vi "#0_MAV_MSG_HEARTBEAT.vi"(11 "mavlink_payload":u8[](array[numeric])) -> (3 "HEARTBEAT":T1)   [LabVIEW 2023]
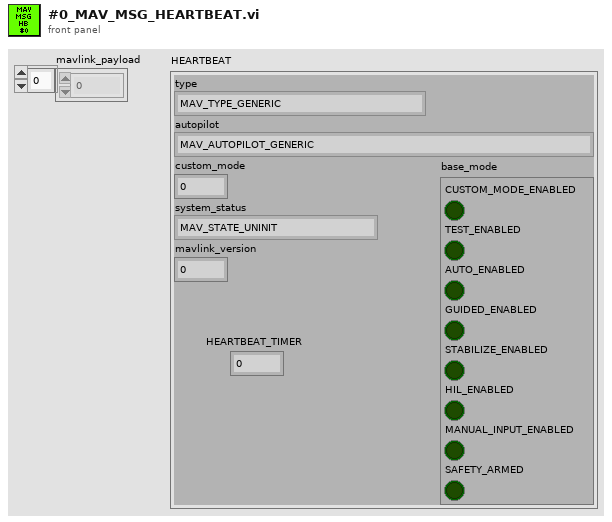
[diagram p1: front panel]
types:
  T1 = cluster{"type":enum8{"MAV_TYPE_GENERIC", "MAV_TYPE_FIXED_WING", "MAV_TYPE_QUADROTOR", "MAV_TYPE_COAXIAL", "MAV_TYPE_HELICOPTER", "MAV_TYPE_ANTENNA_TRACKER", "MAV_TYPE_GCS", "MAV_TYPE_AIRSHIP", "MAV_TYPE_FREE_BALLOON", "MAV_TYPE_ROCKET", "MAV_TYPE_GROUND_ROVER", "MAV_TYPE_SURFACE_BOAT", "MAV_TYPE_SUBMARINE", "MAV_TYPE_HEXAROTOR", "MAV_TYPE_OCTOROTOR", "MAV_TYPE_TRICOPTER", "MAV_TYPE_FLAPPING_WING", "MAV_TYPE_KITE", "MAV_TYPE_ONBOARD_CONTROLLER", "MAV_TYPE_VTOL_TAILSITTER_DUOROTOR", "MAV_TYPE_VTOL_TAILSITTER_QUADROTOR", "MAV_TYPE_VTOL_TILTROTOR", "MAV_TYPE_VTOL_FIXEDROTOR", "MAV_TYPE_VTOL_TAILSITTER", "MAV_TYPE_VTOL_TILTWING", "MAV_TYPE_VTOL_RESERVED5", "MAV_TYPE_GIMBAL", "MAV_TYPE_ADSB", "MAV_TYPE_PARAFOIL", "MAV_TYPE_DODECAROTOR", "MAV_TYPE_CAMERA", "MAV_TYPE_CHARGING_STATION", "MAV_TYPE_FLARM", "MAV_TYPE_SERVO", "MAV_TYPE_ODID", "MAV_TYPE_DECAROTOR", "MAV_TYPE_BATTERY", "MAV_TYPE_PARACHUTE", "MAV_TYPE_LOG", "MAV_TYPE_OSD", "MAV_TYPE_IMU", "MAV_TYPE_GPS", "MAV_TYPE_WINCH", "MAV_TYPE_GENERIC_MULTIROTOR", "MAV_TYPE_ILLUMINATOR"}, "autopilot":enum8{"MAV_AUTOPILOT_GENERIC", "MAV_AUTOPILOT_RESERVED", "MAV_AUTOPILOT_SLUGS", "MAV_AUTOPILOT_ARDUPILOTMEGA", "MAV_AUTOPILOT_OPENPILOT", "MAV_AUTOPILOT_GENERIC_WAYPOINTS_ONLY", "MAV_AUTOPILOT_GENERIC_WAYPOINTS_AND_SIMPLE_NAVIGATION_ONLY", "MAV_AUTOPILOT_GENERIC_MISSION_FULL", "MAV_AUTOPILOT_INVALID", "MAV_AUTOPILOT_PPZ", "MAV_AUTOPILOT_UDB", "MAV_AUTOPILOT_FP", "MAV_AUTOPILOT_PX4", "MAV_AUTOPILOT_SMACCMPILOT", "MAV_AUTOPILOT_AUTOQUAD", "MAV_AUTOPILOT_ARMAZILA", "MAV_AUTOPILOT_AEROB", "MAV_AUTOPILOT_ASLUAV", "MAV_AUTOPILOT_SMARTAP", "MAV_AUTOPILOT_AIRRAILS", "MAV_AUTOPILOT_REFLEX"}, "custom_mode":u32, "system_status":enum16{"MAV_STATE_UNINIT", "MAV_STATE_BOOT", "MAV_STATE_CALIBRATING", "MAV_STATE_STANDBY", "MAV_STATE_ACTIVE", "MAV_STATE_CRITICAL", "MAV_STATE_EMERGENCY", "MAV_STATE_POWEROFF", "MAV_STATE_FLIGHT_TERMINATION"}, "mavlink_version":u8, "base_mode":cluster{"CUSTOM_MODE_ENABLED":bool, "TEST_ENABLED":bool, "AUTO_ENABLED":bool, "GUIDED_ENABLED":bool, "STABILIZE_ENABLED":bool, "HIL_ENABLED":bool, "MANUAL_INPUT_ENABLED":bool, "SAFETY_ARMED":bool}, "HEARTBEAT_TIMER":u32}
  T2 = enum16{"MAV_STATE_UNINIT", "MAV_STATE_BOOT", "MAV_STATE_CALIBRATING", "MAV_STATE_STANDBY", "MAV_STATE_ACTIVE", "MAV_STATE_CRITICAL", "MAV_STATE_EMERGENCY", "MAV_STATE_POWEROFF", "MAV_STATE_FLIGHT_TERMINATION"}
  T3 = enum8{"MAV_AUTOPILOT_GENERIC", "MAV_AUTOPILOT_RESERVED", "MAV_AUTOPILOT_SLUGS", "MAV_AUTOPILOT_ARDUPILOTMEGA", "MAV_AUTOPILOT_OPENPILOT", "MAV_AUTOPILOT_GENERIC_WAYPOINTS_ONLY", "MAV_AUTOPILOT_GENERIC_WAYPOINTS_AND_SIMPLE_NAVIGATION_ONLY", "MAV_AUTOPILOT_GENERIC_MISSION_FULL", "MAV_AUTOPILOT_INVALID", "MAV_AUTOPILOT_PPZ", "MAV_AUTOPILOT_UDB", "MAV_AUTOPILOT_FP", "MAV_AUTOPILOT_PX4", "MAV_AUTOPILOT_SMACCMPILOT", "MAV_AUTOPILOT_AUTOQUAD", "MAV_AUTOPILOT_ARMAZILA", "MAV_AUTOPILOT_AEROB", "MAV_AUTOPILOT_ASLUAV", "MAV_AUTOPILOT_SMARTAP", "MAV_AUTOPILOT_AIRRAILS", "MAV_AUTOPILOT_REFLEX"}
  T4 = enum8{"MAV_TYPE_GENERIC", "MAV_TYPE_FIXED_WING", "MAV_TYPE_QUADROTOR", "MAV_TYPE_COAXIAL", "MAV_TYPE_HELICOPTER", "MAV_TYPE_ANTENNA_TRACKER", "MAV_TYPE_GCS", "MAV_TYPE_AIRSHIP", "MAV_TYPE_FREE_BALLOON", "MAV_TYPE_ROCKET", "MAV_TYPE_GROUND_ROVER", "MAV_TYPE_SURFACE_BOAT", "MAV_TYPE_SUBMARINE", "MAV_TYPE_HEXAROTOR", "MAV_TYPE_OCTOROTOR", "MAV_TYPE_TRICOPTER", "MAV_TYPE_FLAPPING_WING", "MAV_TYPE_KITE", "MAV_TYPE_ONBOARD_CONTROLLER", "MAV_TYPE_VTOL_TAILSITTER_DUOROTOR", "MAV_TYPE_VTOL_TAILSITTER_QUADROTOR", "MAV_TYPE_VTOL_TILTROTOR", "MAV_TYPE_VTOL_FIXEDROTOR", "MAV_TYPE_VTOL_TAILSITTER", "MAV_TYPE_VTOL_TILTWING", "MAV_TYPE_VTOL_RESERVED5", "MAV_TYPE_GIMBAL", "MAV_TYPE_ADSB", "MAV_TYPE_PARAFOIL", "MAV_TYPE_DODECAROTOR", "MAV_TYPE_CAMERA", "MAV_TYPE_CHARGING_STATION", "MAV_TYPE_FLARM", "MAV_TYPE_SERVO", "MAV_TYPE_ODID", "MAV_TYPE_DECAROTOR", "MAV_TYPE_BATTERY", "MAV_TYPE_PARACHUTE", "MAV_TYPE_LOG", "MAV_TYPE_OSD", "MAV_TYPE_IMU", "MAV_TYPE_GPS", "MAV_TYPE_WINCH", "MAV_TYPE_GENERIC_MULTIROTOR", "MAV_TYPE_ILLUMINATOR"}
  T5 = cluster{"Boolean array[0]":bool, "Boolean array[1]":bool, "Boolean array[2]":bool, "Boolean array[3]":bool, "Boolean array[4]":bool, "Boolean array[5]":bool, "Boolean array[6]":bool, "Boolean array[7]":bool}
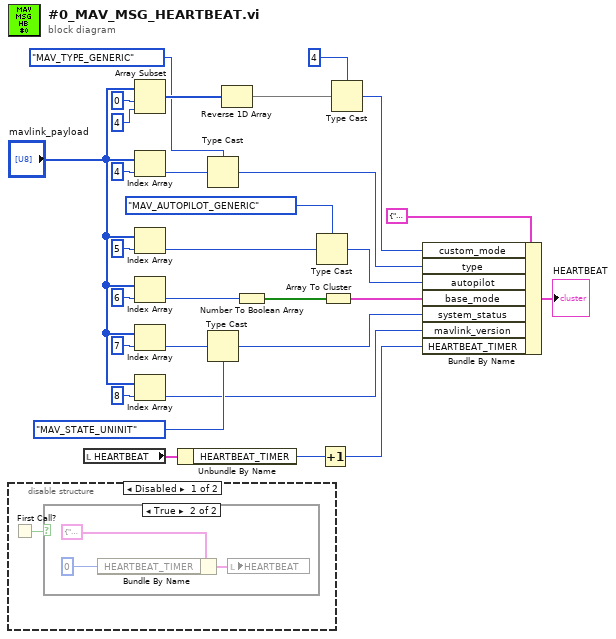
[diagram p0: block diagram]
diagram:
  n1 = disable-structure shown="Disabled" {
    frame Disabled {
      n2 = First Call?() -> (First Call?: T/F=w31:bool)
      n3 = case shown="True" w31 {
        frame False {
        }
        frame True {
          n4 = Bundle By Name(cluster=T1 {"type"=enum."MAV_TYPE_GENERIC", "autopilot"=enum."MAV_AUTOPILOT_GENERIC", "custom_mode"=0, "system_status"=enum."MAV_STATE_UNINIT", "mavlink_version"=0, "base_mode"={"CUSTOM_MODE_ENABLED"=FALSE, "TEST_ENABLED"=FALSE, "AUTO_ENABLED"=FALSE, "GUIDED_ENABLED"=FALSE, "STABILIZE_ENABLED"=FALSE, "HIL_ENABLED"=FALSE, "MANUAL_INPUT_ENABLED"=FALSE, "SAFETY_ARMED"=FALSE}, "HEARTBEAT_TIMER"=0} ("HEARTBEAT"), "HEARTBEAT_TIMER"=u32 0) -> (w34:T1)
          n5 = local write "HEARTBEAT"(w34) -> ()
        }
      }
    }
    frame Enabled {
    }
  }
  n6 = local read "HEARTBEAT"() -> (w8:T1)
  n7 = Array Subset(array="mavlink_payload", index=0, length=4) -> (w30:u8[])
  n8 = Index Array(array="mavlink_payload", index=4) -> (element=w26:u8)
  n9 = Index Array(array="mavlink_payload", index=5) -> (element=w23:u8)
  n10 = Index Array(array="mavlink_payload", index=6) -> (element=w3:u8)
  n11 = Index Array(array="mavlink_payload", index=7) -> (element=w14:u8)
  n12 = Index Array(array="mavlink_payload", index=8) -> (element=w9:u8)
  n13 = Unbundle By Name(w8) -> ("HEARTBEAT_TIMER"=w7:u32)
  n14 = Type Cast(type=T4."MAV_TYPE_GENERIC", x=w26) -> (*(type *) &x=w24:T4)
  n15 = Type Cast(type=T2."MAV_STATE_UNINIT" ("system_status"), x=w14) -> (*(type *) &x=w12:T2)
  n16 = Reverse 1D Array(array=w30) -> (reversed array=w29:u8[])
  n17 = Number To Boolean Array(number=w3) -> (Boolean array=w1:bool[])
  n18 = Type Cast(type=T3."MAV_AUTOPILOT_GENERIC" ("autopilot"), x=w23) -> (*(type *) &x=w22:T3)
  n19 = Increment(x=w7) -> (x+1=w6:u32)
  n20 = Array To Cluster(array=w1) -> (cluster=w2:T5)
  n21 = Type Cast(type=u32 4 ("index"), x=w29) -> (*(type *) &x=w16:u32)
  n22 = Bundle By Name(cluster=T1 {"type"=enum."MAV_TYPE_GENERIC", "autopilot"=enum."MAV_AUTOPILOT_GENERIC", "custom_mode"=0, "system_status"=enum."MAV_STATE_UNINIT", "mavlink_version"=0, "base_mode"={"CUSTOM_MODE_ENABLED"=FALSE, "TEST_ENABLED"=FALSE, "AUTO_ENABLED"=FALSE, "GUIDED_ENABLED"=FALSE, "STABILIZE_ENABLED"=FALSE, "HIL_ENABLED"=FALSE, "MANUAL_INPUT_ENABLED"=FALSE, "SAFETY_ARMED"=FALSE}, "HEARTBEAT_TIMER"=0} ("HEARTBEAT"), "custom_mode"=w16, "type"=w24, "autopilot"=w22, "base_mode"=w2, "system_status"=w12, "mavlink_version"=w9, "HEARTBEAT_TIMER"=w6) -> (→"HEARTBEAT":T1)
